vi "ParseError.vi"(8 "error in (no error)":errorcluster, 10 "error":errorcluster, 11 "SimpleErrorLogger in":refnum<class "SimpleErrorLogger.lvclass">) -> (0 "error out":errorcluster, 1 "Code":i32, 2 "TypeOfError":T1, 3 "SimpleErrorLogger out":refnum<class "SimpleErrorLogger.lvclass">, 4 "Message":string, 5 "source":string)   [LabVIEW 2023, in "SimpleErrorLogger.lvlib" / "SimpleErrorLogger.lvclass"]
uses:
  SimpleErrorLogger.lvclass
  SimpleErrorLogger.lvclass/SimpleErrorLogger.ctl
  <vilib>/Utility/error.llb/DialogType.ctl
  TypeDefinitions/ErrorType.ctl
  SimpleErrorLogger.lvlib
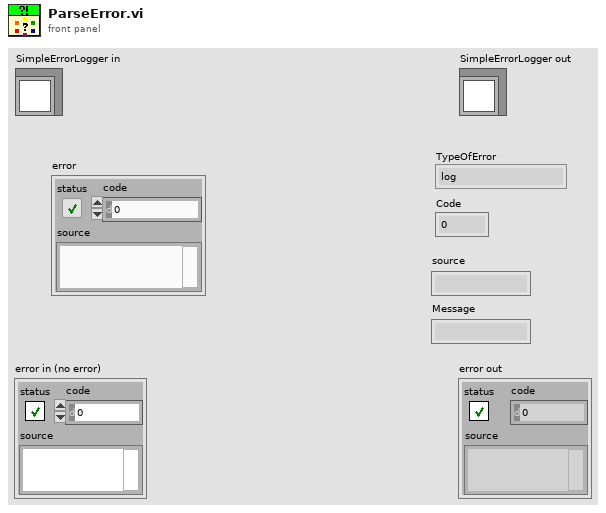
[diagram p1: front panel]
types:
  T1 = typedef "SimpleErrorLogger.lvlib/ErrorType.ctl" = enum16{"log", "fatal", "ignor"}
  T2 = typedef "DialogType.ctl" = u16
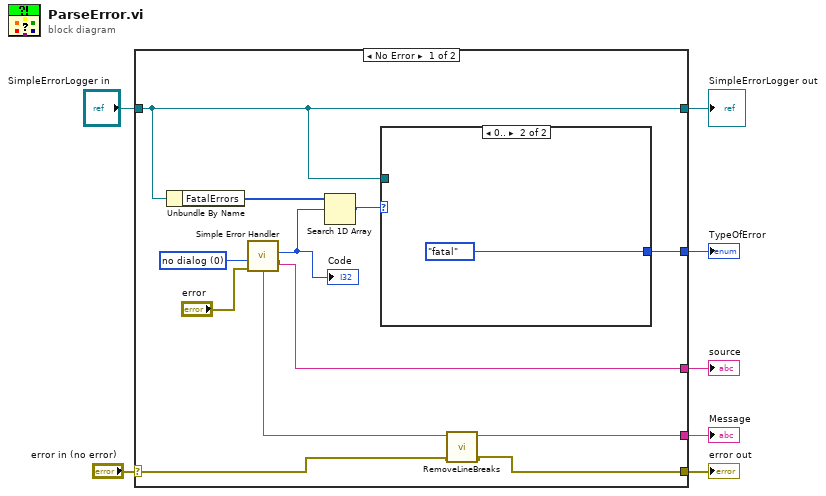
[diagram p0: block diagram]
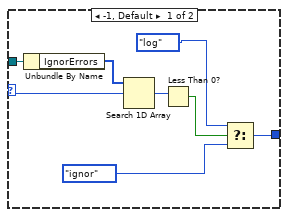
[diagram p2: hidden frame]
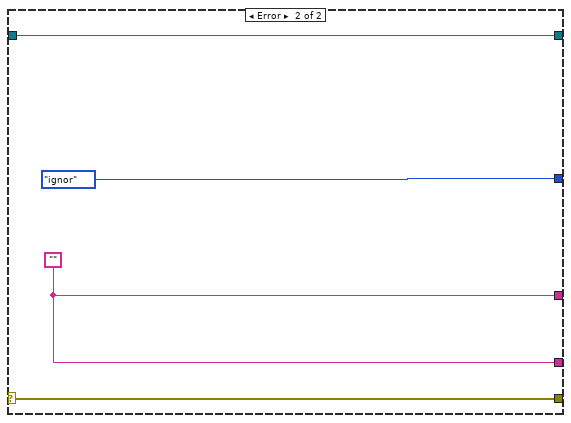
[diagram p3: hidden frame]
diagram:
  n1 = case shown="No Error" "error in (no error)" {
    selector: "error in (no error)" -> [w10 w32]
    tunnel: [w9 w32] -> w6
    tunnel: [w14 w31] -> w4
    tunnel: "SimpleErrorLogger in" -> [w14 w31]
    tunnel: [w15 ErrorType."ignor" ("TypeOfError")] -> w3
    tunnel: [w13 w29] -> w2
    tunnel: [w11 w29] -> w1
    frame No Error {
      w18 = T2 0 items=["no dialog", "OK message", "continue or stop message", "OK message + warnings", "continue/stop + warnings"] ("type of dialog (OK msg:1)")
      n2 = Unbundle By Name(w14) -> ("FatalErrors"=w17:i32[])
      n3 = call <vilib>:"Simple Error Handler.vi"("type of dialog (OK msg:1)"=w18, "error in (no error)"="error") -> ("code out"=w8:i32, "source out"=w13:string, "message"=w12:string)  [unwired: 3 in, 2 out]
      "Code" <- w8
      n4 = Search 1D Array(1D array=w17, element=w8) -> (index of element=w16:i32)  [unwired: 1 in]
      n5 = case shown="0.." w16 {
        selector: w16 -> [w25 _]
        tunnel: [w20 ErrorType."fatal" ("TypeOfError")] -> w15
        tunnel: w14 -> [w27 _]
        frame -1, Default {
          n6 = Unbundle By Name(w27) -> ("IgnorErrors"=w26:i32[])
          n7 = Search 1D Array(1D array=w26, element=w25) -> (index of element=w24:i32)  [unwired: 1 in]
          n8 = Less Than 0?(x=w24) -> (x < 0?=w23:bool)
          n9 = Select(t=ErrorType."log" ("TypeOfError"), s=w23, f=ErrorType."ignor" ("TypeOfError")) -> (s? t:f=w20:T1)
        }
        frame 0.. {
        }
      }
      n10 = call "RemoveLineBreaks.vi"("error in (no error)"=w10, "Input string"=w12) -> ("error out"=w9:errorcluster, "String linefeeds removed"=w11:string)  [unwired: 8 in]
    }
    frame Error {
      w29 = ""
    }
  }
  "error out" <- w6
  "SimpleErrorLogger out" <- w4
  "TypeOfError" <- w3
  "source" <- w2
  "Message" <- w1
